vi "Update.vi"(8 "error constant":errorcluster, 9 "Controls":T1, 10 "Zone Setup Array":T2[](array[typedef]), 11 "Index Zone in":i32) -> (0 "error constant 2":errorcluster, 2 "Zone Indicators":T4, 3 "Index Zone out":i32)   [LabVIEW 2016]
doc: "Update de zone indicator (diode and timer)."
uses:
  Controls/Zone Indicators.ctl
  Controls/Zone Setup.ctl
  Controls/Zone.ctl
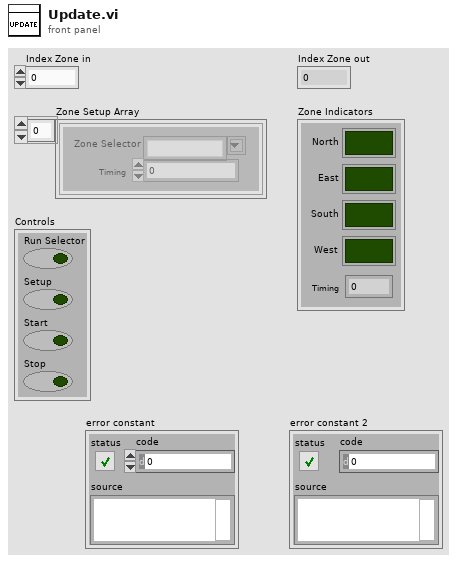
[diagram p1: front panel]
types:
  T1 = cluster{"Run Selector":bool, "Setup":bool, "Start":bool, "Stop":bool}
  T2 = typedef "Zone Setup.ctl" = cluster{"Zone Selector":T3, "Timing":u32}
  T3 = typedef "Zone.ctl" = string
  T4 = typedef "Zone Indicators.ctl" = cluster{"North":bool, "East":bool, "South":bool, "West":bool, "Timing":dbl}
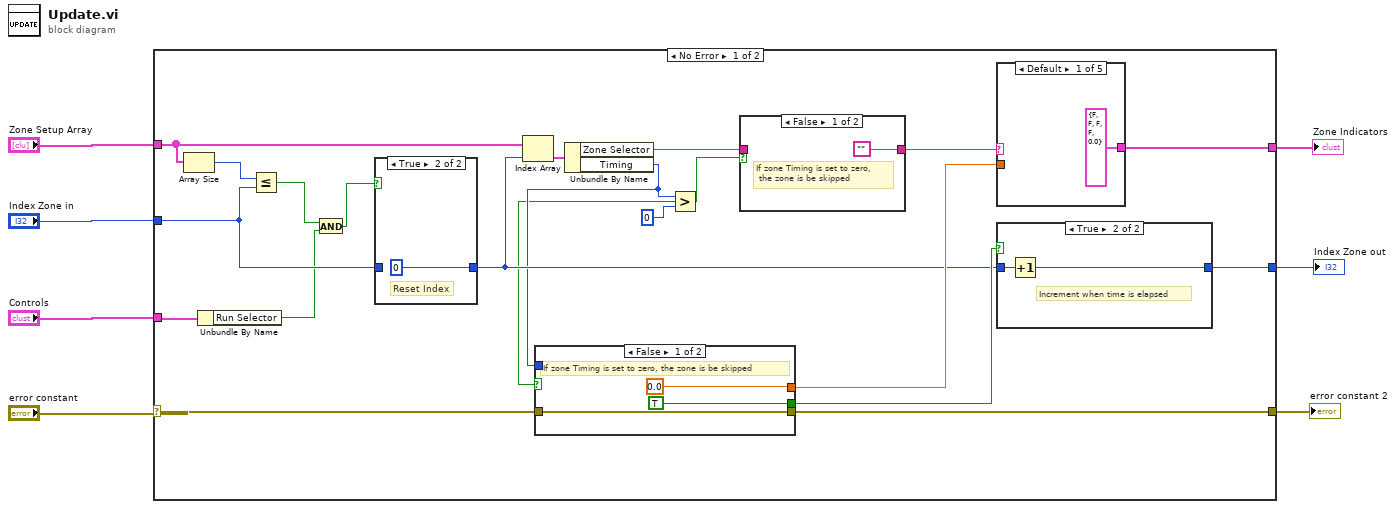
[diagram p0: block diagram]
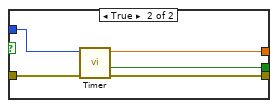
[diagram p3: hidden frame]
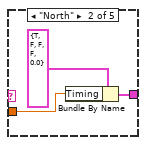
[diagram p5: hidden frame]
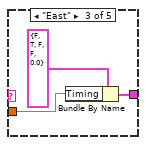
[diagram p6: hidden frame]
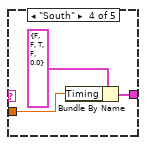
[diagram p7: hidden frame]
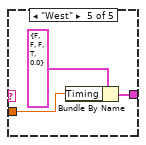
[diagram p8: hidden frame]
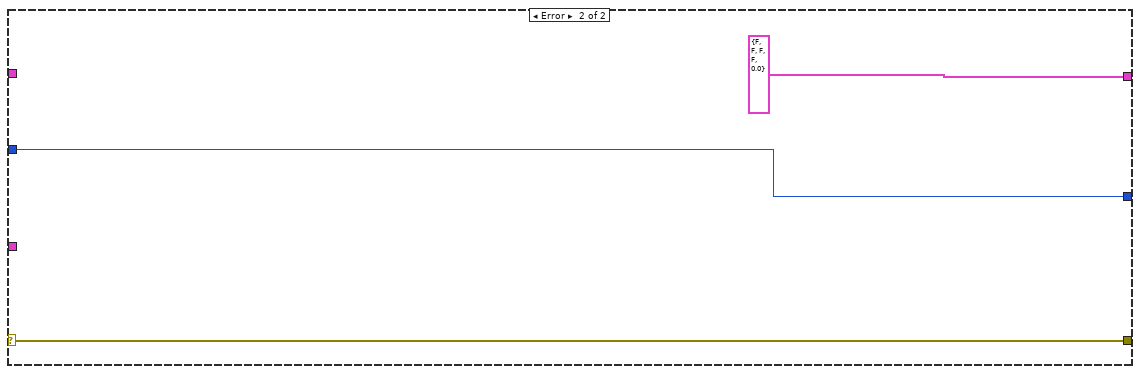
[diagram p10: hidden frame]
diagram:
  n1 = case shown="No Error" "error constant" {
    selector: "error constant" -> [w19 w58]
    tunnel: [w24 w57] -> w7
    tunnel: [w23 T4 {"North"=FALSE, "East"=FALSE, "South"=FALSE, "West"=FALSE, "Timing"=0.0} ("Zone Indicators")] -> w6
    tunnel: "Zone Setup Array" -> [w21 _]
    tunnel: "Index Zone in" -> [w16 w57]
    tunnel: "Controls" -> [w20 _]
    tunnel: [w18 w58] -> w1
    frame No Error {
      n2 = Array Size(array=w21) -> (size(s)=w17:i32)
      n3 = Unbundle By Name(w20) -> ("Run Selector"=w14:bool)
      n4 = Less Or Equal?(x=w17, y=w16) -> (x <= y?=w15:bool)
      n5 = And(x=w15, y=w14) -> (x .and. y?=w13:bool)
      n6 = case shown="True" w13 {
        tunnel: [w54 0 ("Index Zone")] -> w25
        tunnel: w16 -> [w54 _]
        frame False {
        }
        frame True {
          # "Reset Index"
        }
      }
      n7 = Index Array(array=w21, index=w25) -> (element=w22:T2)
      n8 = Unbundle By Name(w22) -> ("Zone Selector"=w9:T3, "Timing"=w11:u32)
      n9 = Greater?(x=w11, y=u32 0) -> (0:w10:bool)
      n10 = case shown="False" w10 {
        tunnel: [0.0 ("Numeric") w37] -> w27
        tunnel: [TRUE ("Time has Elapsed") w36] -> w26
        tunnel: w19 -> [w32 w35]
        tunnel: [w32 w34] -> w18
        tunnel: w11 -> [_ w33]
        frame False {
          # "If zone Timing is set to zero, the zone is be skipped"
        }
        frame True {
          n11 = call "Timer.vi"("error constant"=w35, "Timing"=w33) -> ("error constant 2"=w34:errorcluster, "Time has Elapsed"=w36:bool, "Numeric"=w37:dbl)  [unwired: 7 in]
        }
      }
      n12 = case shown="False" w10 {
        tunnel: w9 -> [_ w29]
        tunnel: ["" w29] -> w8
        frame False {
          # "If zone Timing is set to zero,\n the zone is be skipped"
        }
        frame True {
        }
      }
      n13 = case shown="Default" w8 {
        tunnel: [T4 {"North"=FALSE, "East"=FALSE, "South"=FALSE, "West"=FALSE, "Timing"=0.0} ("Zone Indicators") w43 w46 w49 w52] -> w23
        tunnel: w27 -> [_ w42 w45 w48 w51]
        frame Default {
        }
        frame "North" {
          n14 = Bundle By Name(cluster=T4 {"North"=TRUE, "East"=FALSE, "South"=FALSE, "West"=FALSE, "Timing"=0.0} ("Zone Indicators"), "Timing"=w42) -> (w43:T4)
        }
        frame "East" {
          n15 = Bundle By Name(cluster=T4 {"North"=FALSE, "East"=TRUE, "South"=FALSE, "West"=FALSE, "Timing"=0.0} ("Zone Indicators"), "Timing"=w45) -> (w46:T4)
        }
        frame "South" {
          n16 = Bundle By Name(cluster=T4 {"North"=FALSE, "East"=FALSE, "South"=TRUE, "West"=FALSE, "Timing"=0.0} ("Zone Indicators"), "Timing"=w48) -> (w49:T4)
        }
        frame "West" {
          n17 = Bundle By Name(cluster=T4 {"North"=FALSE, "East"=FALSE, "South"=FALSE, "West"=TRUE, "Timing"=0.0} ("Zone Indicators"), "Timing"=w51) -> (w52:T4)
        }
      }
      n18 = case shown="True" w26 {
        tunnel: [w38 w40] -> w24
        tunnel: w25 -> [w38 w39]
        frame False {
        }
        frame True {
          # "Increment when time is elapsed"
          n19 = Increment(x=w39) -> (x+1=w40:i32)
        }
      }
    }
    frame Error {
    }
  }
  "Index Zone out" <- w7
  "Zone Indicators" <- w6
  "error constant 2" <- w1
